vi "epoch convertor.vi"() -> ()   [LabVIEW 2022 SP3]
panel:
  out "decimal integer string 3":string
  in  "x 2":timestamp=timestamp(2082844800 s since 1904-01-01)
  out "time stamp 2":timestamp
  out "time stamp":timestamp
  out "double precision float":dbl
  out "x-y":dbl
  out "decimal integer string 2":string
  in  "x":timestamp=timestamp(2082844800 s since 1904-01-01)
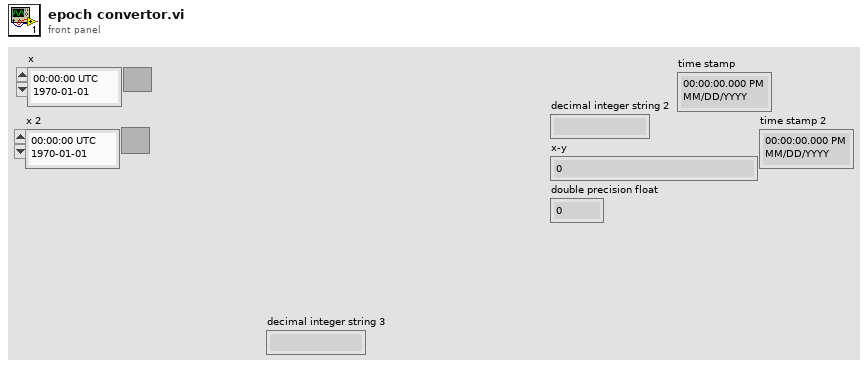
[diagram p1: front panel]
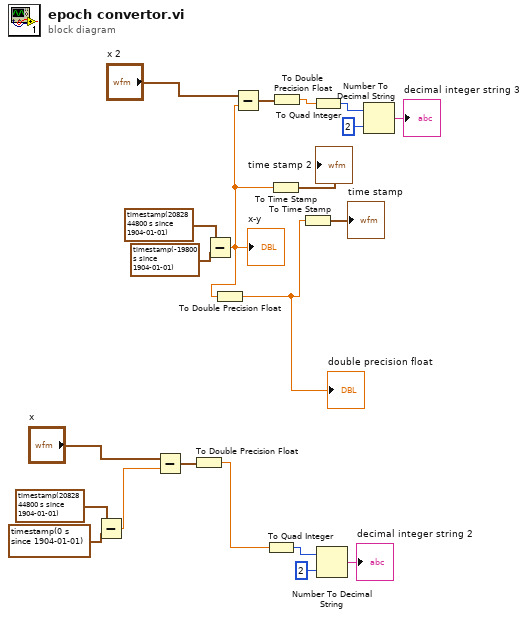
[diagram p0: block diagram]
diagram:
  n1 = Subtract(x=timestamp(2082844800 s since 1904-01-01), y=timestamp(0 s since 1904-01-01) ("current time")) -> (x-y=w20:dbl)
  n2 = Subtract(x="x", y=w20) -> (x-y=w19:timestamp)
  n3 = To Double Precision Float(number=w19) -> (double precision float=w13:dbl)
  n4 = Subtract(x=timestamp(2082844800.001 s since 1904-01-01), y=timestamp(-19799.999 s since 1904-01-01) ("current time")) -> (x-y=w5:dbl)
  "x-y" <- w5
  n5 = To Double Precision Float(number=w5) -> (double precision float=w10:dbl)
  "double precision float" <- w10
  n6 = Subtract(x="x 2", y=w5) -> (x-y=w6:timestamp)
  n7 = To Quad Integer(1:w13) -> (0:w14:i64)
  n8 = To Time Stamp(1:w5) -> (0:→"time stamp 2":timestamp)
  n9 = To Double Precision Float(number=w6) -> (double precision float=w1:dbl)
  n10 = To Time Stamp(1:w10) -> (0:→"time stamp":timestamp)
  n11 = To Quad Integer(1:w1) -> (0:w4:i64)
  n12 = Number To Decimal String(number=w14, width (-)=i16 2) -> (decimal integer string=→"decimal integer string 2":string)
  n13 = Number To Decimal String(number=w4, width (-)=i16 2) -> (decimal integer string=→"decimal integer string 3":string)
